vi "TIFF_Cluster_to_Json.vi"() -> ()   [LabVIEW 2025]
uses:
  TypeDef_Array_ChannelCluster.ctl
  <vilib>/addons/_JKI.lib/Serialization/JSON/JKI JSON Serialization.lvlib
panel:
  in  "Channel_Cluster_Array":T1=[{"Laser"=enum."640 nm", "Power"=90, "Exposure time"=0.05, "Channel ON-OFF"=TRUE, "Polar ON-OFF"=TRUE, "FW 1"=0, "FW 2"=0}, {"Laser"=enum."640 nm", "Power"=50, "Exposure time"=0.05, "Channel ON-OFF"=FALSE, "Polar ON-OFF"=FALSE, "FW 1"=0, "FW 2"=0}, {"Laser"=enum."640 nm", "Power"=20, "Exposure time"=0.05, "Channel ON-OFF"=FALSE, "Polar ON-OFF"=FALSE, "FW 1"=0, "FW 2"=0}] {"FW 2" items=["447/60", "475/35", "525/50", "600/37", "647/37", "647LP"]; "FW 1" items=["447/60", "475/35", "525/50", "600/37", "647/57", "647LP"]; "Exposure time" min=0.0 max=5.0 step=0.01; "Power" max=100 step=1}
  out "JSON String":string
  in  "error in (no error)":errorcluster
  out "error out":errorcluster
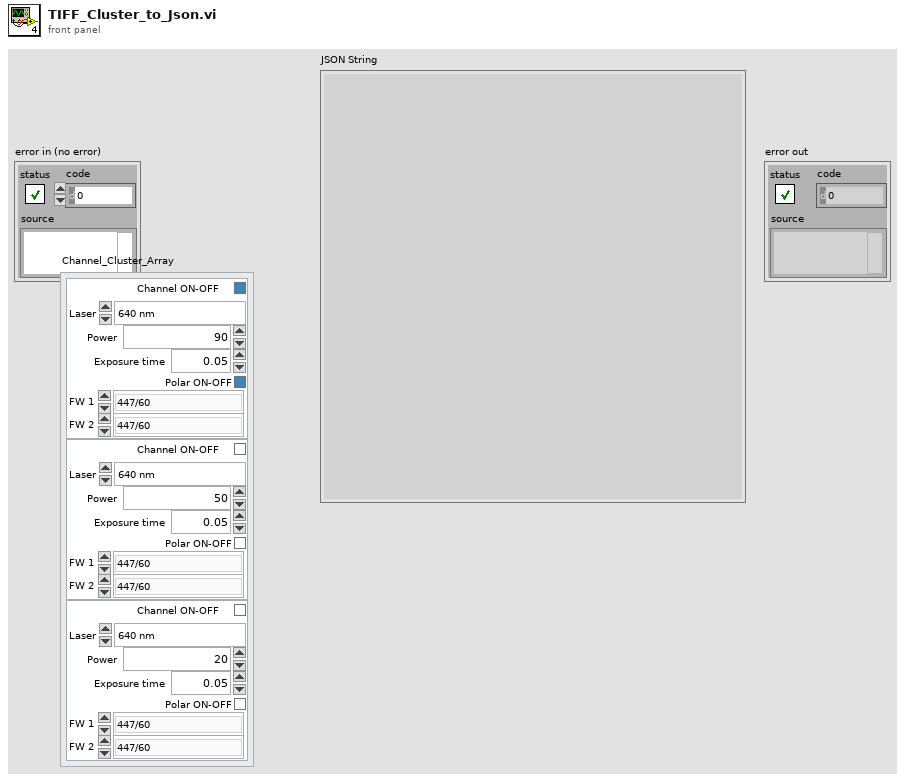
[diagram p1: front panel]
types:
  T1 = typedef "TypeDef_Array_ChannelCluster.ctl" = cluster{"Laser":enum16{"640 nm", "561 nm"}, "Power":u8, "Exposure time":dbl, "Channel ON-OFF":bool, "Polar ON-OFF":bool, "FW 1":u16, "FW 2":u16}[]
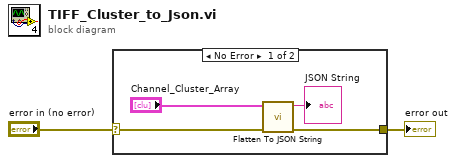
[diagram p0: block diagram]
diagram:
  n1 = case shown="No Error" "error in (no error)" {
    selector: "error in (no error)" -> [w6 w7]
    tunnel: [w4 w7] -> w2
    frame No Error {
      n2 = call <vilib>:"Flatten To JSON String.vi"("error in"=w6, "Variant"="Channel_Cluster_Array") -> ("error out"=w4:errorcluster, "JSON String"=→"JSON String":string)  [unwired: 8 in]
    }
    frame Error {
    }
  }
  "error out" <- w2
